vi "cp.vi"(0 "IP adress":string="192.109.209.229", 1 "stop":bool, 2 "Channel":u8(ring) items=["1", "2", "3", "4", "5", "6", "7", "8", "9", "10", "11", "12", "13", "14", "15", "16"], 3 "CP Parameters":T1={"Steps"=[{"vs_initial"=FALSE, "Current_step"=0.0, "Duration_step"=1.0}, {"vs_initial"=FALSE, "Current_step"=0.001, "Duration_step"=1.0}, {"vs_initial"=FALSE, "Current_step"=0.005, "Duration_step"=1.0}], "Step_number"=2, "N_Cycles"=0, "Record_every_dE"=0.005, "Record_every_dT"=0.05, "I_Range"=8, "E_Range"=3, "Bandwidth"=5, "em"=1, "ce"=0, "tb"=2.5e-05} {"tb" min=2.5e-05 max=1 format="%^_3e"; "ce" items=["Standard", "CE to ground"]; "N_Cycles" min=0 max=1000000; "Step_number" min=0 max=99; "E_Range" items=["±2.5V", "±5V", "±10V", "Auto"]; "Bandwidth" items=["1"=1, "2"=2, "3"=3, "4"=4, "5"=5, "6"=6, "7"=7, "8"=8, "9"=9]; "Record_every_dT" min=0.0001 max=1000 format="%^_3e"; "Record_every_dE" format="%^_3e"; "I_Range" items=["1pA", "1nA", "10nA", "100nA", "1µA", "10µA", "100µA", "1mA", "10mA", "100mA", "1A", "Booster"]; "Steps"."Duration_step" min=0.001 max=80000 format="%^_3e"; "Steps"."Current_step" min=-150 max=150 format="%^_3e"}, 4 "Exit":bool, 5 "Start":bool, 6 "Draw":enum16{"Ewe(t)", "I(t)"}(ring)) -> (7 "XY Graph":cluster{"Data 101":sgl[], "Data 101":sgl[]}(graph), 8 "Number of points":i32=5992)   [LabVIEW 2012]
doc: "The Chrono-Potentiometry (CP) is a controlled current technique. The current is controlled and the potential is the variable determined as a function of time.\nIn general, in this VI, the first thing to do is to start by establishing the connection with the instrument defined by its IP adress, then load the firmware in the channel selected, get the information on the plugged channels, load protocol on a channel, start/stop the protocol, retreive data and draw the graph."
uses:
  base_xml.llb/Type Descriptor Enumeration__ogtk.ctl
panel:
  out "Exit 2":bool=TRUE
  out "Data 102":sgl[][](array[numeric]) format="%.2f"
  # "Instructions:\nBefore running the VI you must type a valid IP adress that corresponds to the instrument.Then press the Run button to execute this VI.\nWhile this VI is running, choose the available channel, enter the CP parameters or keep the default values, then press the start button to begin the experience.\nChoose the waveform to draw (Ewe(t) or I(t)). You can stop the measure if you press the stop button and exit the execution if you press the exit button."
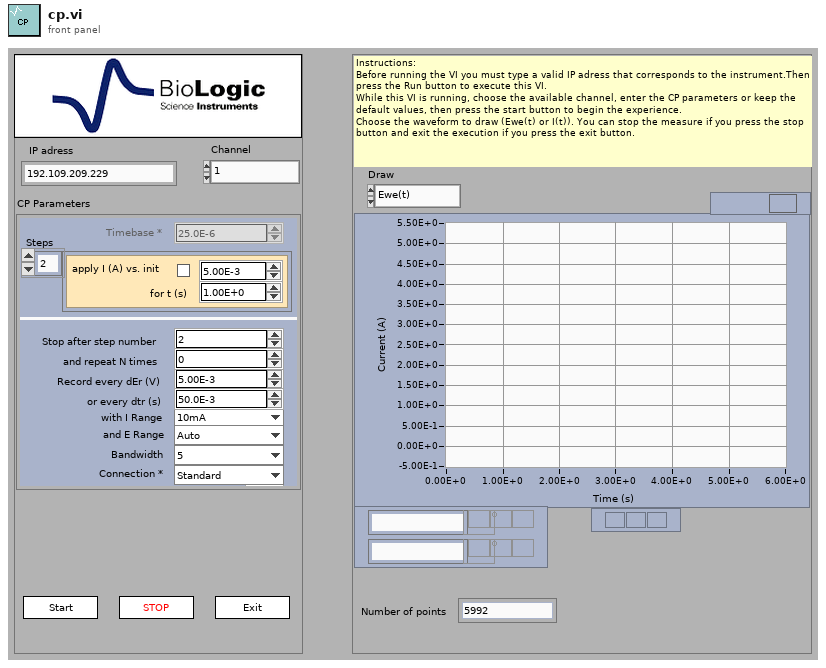
[diagram p1: front panel]
types:
  T1 = cluster{"Steps":cluster{"vs_initial":bool, "Current_step":sgl, "Duration_step":sgl}[], "Step_number":i32, "N_Cycles":i32, "Record_every_dE":sgl, "Record_every_dT":sgl, "I_Range":u16, "E_Range":u16, "Bandwidth":u16, "em":u16, "ce":u16, "tb":sgl}
  T2 = typedef "Type Descriptor Enumeration__ogtk.ctl" = enum8{"<Null>", "I8", "I16", "I32", "I64", "U8", "U16", "U32", "U64", "SGL", "DBL", "EXT", "CSG", "CDB", "CXT", "0x0F", "0x10", "0x11", "0x12", "0x13", "0x14", "Enum U8", "Enum U16", "Enum U32", "Enum U64", "SGL PQ", "DBL PQ", "EXT PQ", "CSG PQ", "CDB PQ", "CXT PQ", "0x1F", "0x20", "Boolean", "0x22", "0x23", "0x24", "0x25", "0x26", "0x27", "0x28", "0x29", "0x2A", "0x2B", "0x2C", "0x2D", "0x2E", "0x2F", "String", "0x31", "Path", "Pict", "0x34", "0x35", "0x36", "DAQ", "0x38", "0x39", "0x3A", "0x3B", "0x3C", "0x3D", "0x3E", "0x3F", "Array", "0x41", "0x42", "0x43", "0x44", "0x45", "0x46", "0x47", "0x48", "0x49", "0x4A", "0x4B", "0x4C", "0x4D", "0x4E", "0x4F", "Cluster", "0x51", "0x52", "Variant", "Waveform", "0x55", "0x56", "0x57", "0x58", "0x59", "0x5A", "0x5B", "0x5C", "0x5D", "0x5E", "0x5F", "0x60", "0x61", "0x62", "0x63", "0x64", "0x65", "0x66", "0x67", "0x68", "0x69", "0x6A", "0x6B", "0x6C", "0x6D", "0x6E", "0x6F", "Refnum"}
  T3 = cluster{"Data Type":T2, "Format String":string}[]
  T4 = cluster{"Channel":i32, "BoardVersion":i32, "BoardSerialCode":i32, "FirmwareCode":i32, "FirmwareVersion":i32, "XilinxVersion":i32, "AmpCode":i32, "NbAmp":i32, "LcBoard":i32, "Zboard":i32, "MuxBoard":i32, "GPRAboard":i32, "MemSize":i32, "MemFilled":i32, "state":i32, "MaxIRange":i32, "MinIRange":i32, "MaxBandwidth":i32, "NbOfTechniques":i32}
  T5 = cluster{"Label":string, "type":i32, "valeur":u32, "index":i32}[]
  T6 = cluster{"IRQskipped":i32, "NbRaws":i32, "NbCols":i32, "Technique Index":i32, "TechniqueID":i32, "PrcessIndex":i32, "loop":i32, "StartTime":dbl, "MuxPad":i32}
  T7 = cluster{"State":i32, "MemFilled":i32, "TimeBase":sgl, " Ewe":sgl, " EweRangeMin":sgl, " EweRangeMax":sgl, "Ece":sgl, "EceRangeMin":sgl, "EceRangeMax":sgl, "Eoverflow":i32, "I":sgl, "IRange":i32, "Ioverflow":i32, "ElapsedTime":sgl, "Freq":sgl, "Rcomp":sgl, "Saturation":sgl, "OptErr":i32, "OptPos":i32}
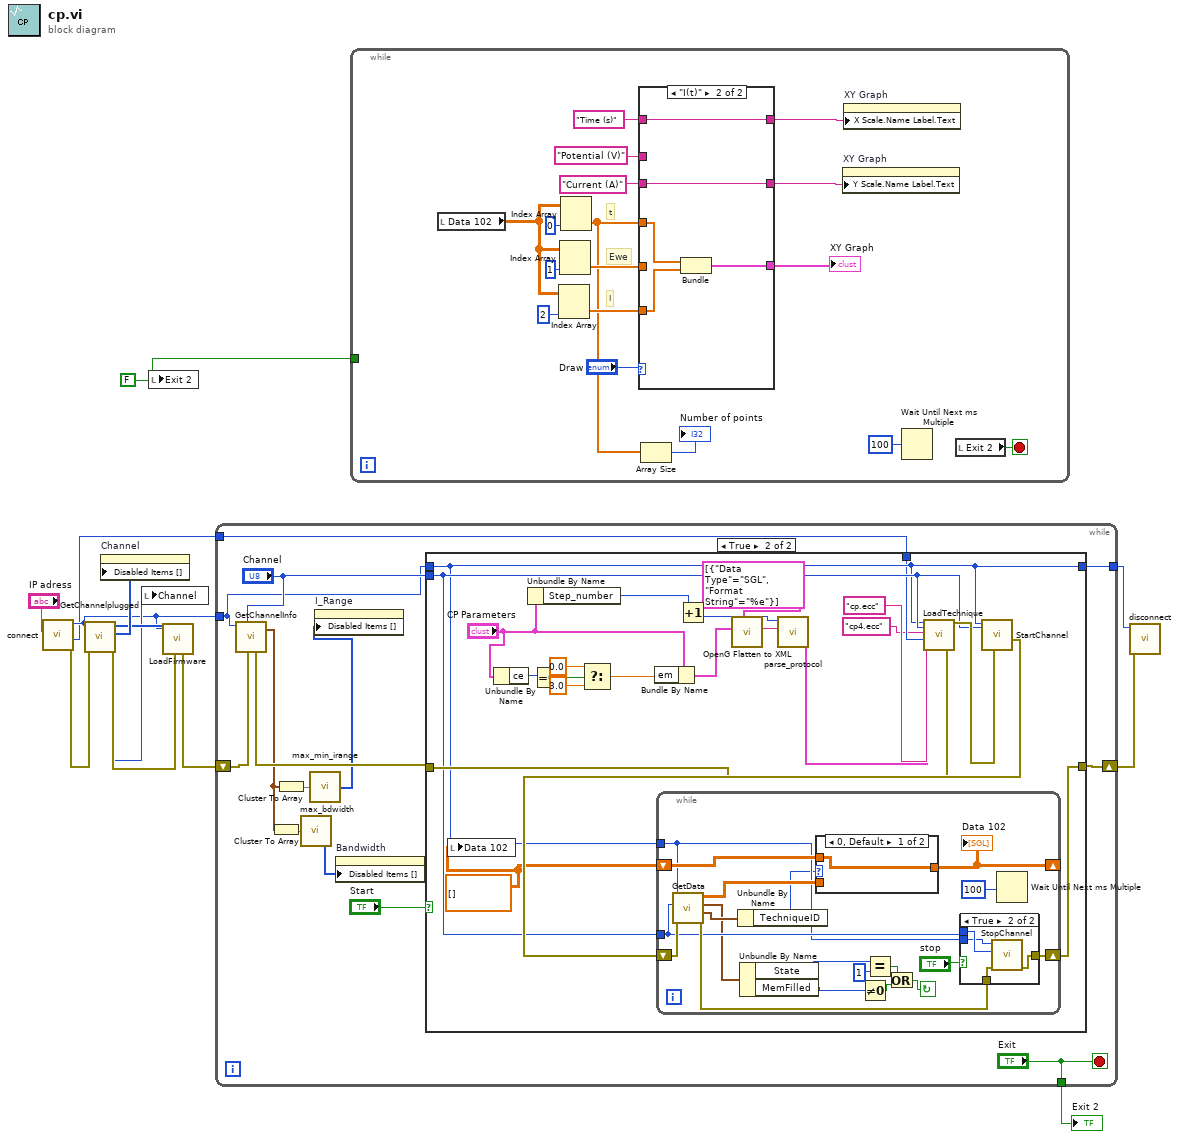
[diagram p0: block diagram]
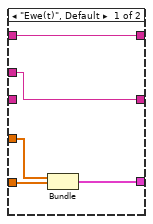
[diagram p2: hidden frame]
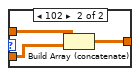
[diagram p5: hidden frame]
diagram:
  w12 = FALSE ("Exit 2")
  n1 = call "connect.vi"("IP"="IP adress") -> ("error out"=w10:errorcluster, "Device Code"=w1:i32, "ID"=w3:i32)  [unwired: 7 in, 1 out]
  n2 = call "GetChannelplugged.vi"("error in (no error)"=w10, "ID"=w3) -> ("error out"=w7:errorcluster, "First channel"=w5:i32, "Disabled channels"=w9:i32[], "Plugged channels"=w8:i32[])  [unwired: 6 in]
  n3 = property on="Channel" class="Ring (strict)"("Disabled Items []"=w9) -> ()  [unwired: 2 in, 2 out]
  n4 = local write "Channel"(w5) -> ()
  n5 = local write "Exit 2"(w12) -> ()
  n6 = call "LoadFirmware.vi"("error in (no error)"=w7, "Channels"=w8, "ID"=w3) -> ("error out"=w4:errorcluster)  [unwired: 7 in, 1 out]
  n7 = while {
    shift-right: [w26] -> w11
    shift-left: w4 -> [w23]
    tunnel: ["Exit"] -> w13
    tunnel: w3 -> [w18]
    tunnel: [w17] -> w2
    tunnel: w1 -> [w14]
    stop <- "Exit" stop-if-true
    n8 = call "GetChannelInfo.vi"("error in (no error)"=w23, "Channel"="Channel", "ID"=w18) -> ("error out"=w22:errorcluster, "Channel information"=w19:T4)  [unwired: 7 in]
    n9 = Cluster To Array(cluster=w19) -> (array=w20:i32[])
    n10 = Cluster To Array(cluster=w19) -> (array=w21:i32[])
    n11 = call "max_bdwidth.vi"("resources"=w20) -> ("disabled ranges"=w15:i32[])
    n12 = call "max_min_irange.vi"("resources"=w21) -> ("disabled ranges"=w16:i32[])
    n13 = property on="I_Range" class="Ring (strict)"("Disabled Items []"=w16) -> ()  [unwired: 2 in, 2 out]
    n14 = property on="Bandwidth" class="Ring (strict)"("Disabled Items []"=w15) -> ()  [unwired: 2 in, 2 out]
    n15 = case shown="True" "Start" {
      tunnel: "Channel" -> [_ w45]
      tunnel: [w29 w48] -> w26
      tunnel: w22 -> [w29 w47]
      tunnel: w18 -> [w28 w41]
      tunnel: [w28 w41] -> w17
      tunnel: w14 -> [_ w38]
      frame False {
      }
      frame True {
        w46 = sgl[][] []
        n16 = local write "Data 102"(w46) -> ()
        n17 = Unbundle By Name("CP Parameters") -> ("ce"=w33:u16)
        n18 = Unbundle By Name("CP Parameters") -> ("Step_number"=w40:i32)
        n19 = Equal To 0?(x=w33) -> (x = 0?=w32:bool)
        n20 = Select(t=0.0, s=w32, f=3.0) -> (s? t:f=w36:dbl)
        n21 = Bundle By Name(cluster="CP Parameters", "em"=w36) -> (w30:T1)
        n22 = Increment(x=w40) -> (x+1=w39:i32)
        n23 = call "OpenG Flatten to XML.vi"("Type Formats (default)"=T3 [{"Data Type"=enum."SGL", "Format String"="%e"}] ("Type Formats"), "LabVIEW Data"=w30) -> ("XML String"=w43:string)  [unwired: 8 in, 1 out]
        n24 = call "parse_protocol.vi"("XML String In"=w43, "index array"=w39) -> ("Params Values"=w42:T5)  [unwired: 7 in]
        n25 = call "LoadTechnique.vi"("ID"=w41, "Selected Channel"=w45, "FName4"="cp4.ecc", "Device Code"=w38, "FName"="cp.ecc", "Protocol Parameters"=w42, "error in (no error)"=w47) -> ("error out"=w50:errorcluster)  [unwired: 12 in]
        n26 = call "StartChannel.vi"("error in (no error)"=w50, "Channel"=w45, "ID"=w41) -> ("error out"=w49:errorcluster)  [unwired: 8 in]
        n27 = while {
          shift-right: [w64] -> w48
          shift-left: w49 -> [w67]
          shift-right: [w61] -> _
          shift-left: w46 -> [w62]
          tunnel: w45 -> [w58]
          tunnel: w41 -> [w57]
          stop <- w65 continue-if-true
          n28 = call "GetData.vi"("error in (no error)"=w67, "Channel"=w58, "ID"=w57) -> ("error out"=w60:errorcluster, "Data information"=w56:T6, "Current values"=w55:T7, "Data"=w63:dbl[][])  [unwired: 5 in]
          n29 = Unbundle By Name(w56) -> ("TechniqueID"=w52:i32)
          n30 = Unbundle By Name(w55) -> ("State"=w54:i32, "MemFilled"=w53:i32)
          n31 = case shown="0, Default" w52 {
            tunnel: w63 -> [_ w79]
            tunnel: w62 -> [w76 w78]
            tunnel: [w76 w77] -> w61
            frame 0, Default {
            }
            frame 102 {
              n32 = Build Array (concatenate)(w78, w79) -> (w77:dbl[][])
            }
          }
          "Data 102" <- w61
          n33 = Not Equal To 0?(x=w53) -> (x != 0?=w68:bool)
          n34 = Equal?(x=w54, y=1) -> (x = y?=w69:bool)
          n35 = Or(x=w69, y=w68) -> (x .or. y?=w65:bool)
          n36 = case shown="True" "stop" {
            tunnel: [w71 w75] -> w64
            tunnel: w60 -> [w71 w74]
            tunnel: w58 -> [_ w73]
            tunnel: w57 -> [_ w72]
            frame False {
            }
            frame True {
              n37 = call "StopChannel.vi"("error in (no error)"=w74, "Channel"=w73, "ID"=w72) -> ("error out"=w75:errorcluster)  [unwired: 8 in]
            }
          }
          n38 = Wait Until Next ms Multiple(millisecond multiple=u32 100) -> ()  [unwired: 1 out]
        }
      }
    }
  }
  "Exit 2" <- w13
  n39 = while {
    tunnel: w12 -> [_]
    stop <- w95 stop-if-true
    # "I"
    # "Ewe"
    # "t"
    n40 = local read "Data 102"() -> (w84:sgl[][])
    n41 = Index Array(array=w84, index (col)=2 ("indice désactivé (col)")) -> (element=w81:sgl[])  [unwired: 1 in]
    n42 = Index Array(array=w84, index (col)=1 ("Index")) -> (element=w83:sgl[])  [unwired: 1 in]
    n43 = Index Array(array=w84, index (col)=0 ("Index")) -> (element=w80:sgl[])  [unwired: 1 in]
    n44 = case shown="\"I(t)\"" "Draw" {
      tunnel: w80 -> [w101 w106]
      tunnel: [w98 w102] -> w82
      tunnel: "Potential (V)" ("Y Scale.Name Label.Text") -> [w100 _]
      tunnel: "Current (A)" ("Y Scale.Name Label.Text") -> [_ w105]
      tunnel: [w100 w105] -> w89
      tunnel: [w99 w104] -> w88
      tunnel: "Time (s)" ("Y Scale.Name Label.Text") -> [w99 w104]
      tunnel: w83 -> [w97 _]
      tunnel: w81 -> [_ w103]
      frame "Ewe(t)", Default {
        n45 = Bundle("Data 102"=w101, "Data 102"=w97) -> (w98:cluster{"Data 102":sgl[], "Data 102":sgl[]})  [unwired: 1 in]
      }
      frame "I(t)" {
        n46 = Bundle("Data 102"=w106, "Data 102"=w103) -> (w102:cluster{"Data 102":sgl[], "Data 102":sgl[]})  [unwired: 1 in]
      }
    }
    "XY Graph" <- w82
    n47 = Array Size(array=w80) -> (size(s)=→"Number of points":i32)
    n48 = property on="XY Graph" class="XYGraph (strict)"("Y Scale.Name Label.Text"=w89) -> ()  [unwired: 2 in, 2 out]
    n49 = property on="XY Graph" class="XYGraph (strict)"("X Scale.Name Label.Text"=w88) -> ()  [unwired: 2 in, 2 out]
    n50 = Wait Until Next ms Multiple(millisecond multiple=u32 100) -> ()  [unwired: 1 out]
    n51 = local read "Exit 2"() -> (w95:bool)
  }
  n52 = call "disconnect.vi"("error in (no error)"=w11, "ID"=w2) -> ()  [unwired: 9 in, 1 out]
